vi "Game of Life.vi"() -> ()   [LabVIEW 2021, in "Game of Life.lvlib"]
doc: "InstrumentStudio plug-in example that displays Conway's Game of Life simulation in a graph."
uses:
  Game of Life.lvlib
  <vilib>/Plug-In SDKs/InstrumentStudio/Plugin Events Enum.ctl
  Helpers/Data Cluster.ctl
  Helpers/Configuration.ctl
  Queue Driver/Queue Operations.ctl
  Queue Driver/Queue State and Data.ctl
  User Event Driver/User Event Operations.ctl
  Helpers/Graph Elements.ctl
  <vilib>/Utility/error.llb/DialogType.ctl
  <vilib>/Utility/error.llb/Error Cluster From Error Code.vi
  <vilib>/ErrorRing/Error Ring.xnode
  <vilib>/Plug-In SDKs/InstrumentStudio/Plugin Session.lvclass
  <vilib>/Plug-In SDKs/InstrumentStudio/InstrumentStudio Plugin SDK.lvlib
  Queue Driver/Queue Driver.lvlib
  User Event Driver/User Event Driver.lvlib
panel:
  in  "Tab Control":enum32{"Game Panel", "Events"}(tab)
  in  "width":u32=100 caption="Board width" min=5 max=1000 step=1
  in  "height":u32=100 caption="Board height" min=5 max=1000 step=1
  in  "update interval":u32=500 caption="Update interval (msec)" min=100 max=2000 step=100
  out "generation":u32 caption="Generation"
  out "game of life":T1(graph)
  in  "Start/Stop":bool
  in  "Log Events?":bool caption="Enable Logging"
  out "Event Record":i32(listbox)=-1
  out "Log file directory":path
  in  "Session Id":u64
  # "When logging is enabled, a log file will be generated in the specified \ndirectory after the front panel is closed."
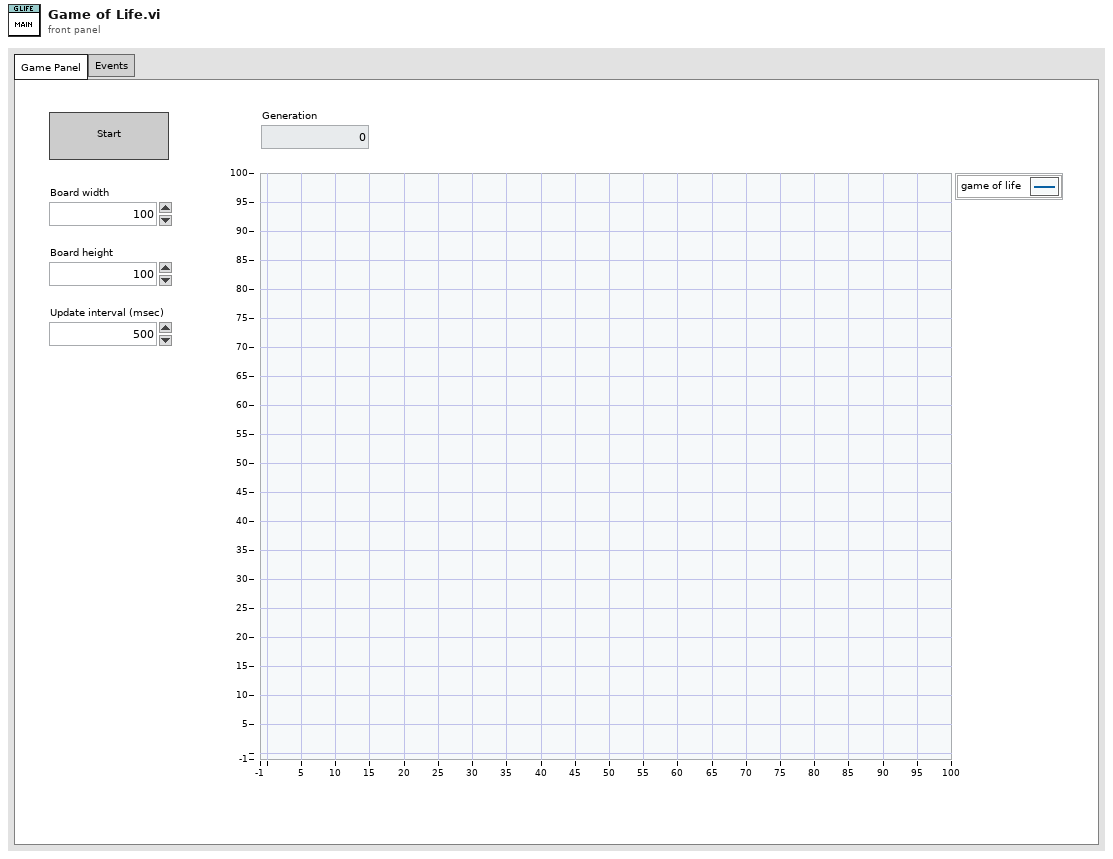
[diagram p1: front panel]
types:
  T1 = typedef "Game of Life.lvlib/Graph Elements.ctl" = cluster{"x data":dbl[], "y data":dbl[]}
  T2 = typedef "Game of Life.lvlib/User Event Driver.lvlib/User Event Operations.ctl" = enum16{"Create", "Destroy", "Get Reference", "Generate"}
  T3 = typedef "Game of Life.lvlib/Queue Driver.lvlib/Queue State and Data.ctl" = cluster{"state":string, "data":variant}
  T4 = typedef "Game of Life.lvlib/Queue Driver.lvlib/Queue Operations.ctl" = enum16{"Create Q", "Enqueue", "Enqueue N", "Enstack", "Enstack N", "Dequeue", "Flush", "Release"}
  T5 = typedef "Game of Life.lvlib/Data Cluster.ctl" = cluster{"configuration":T6, "generation":u32, "cells":bool[][], "event records":string[], "running?":bool, "board update time":timestamp}
  T6 = typedef "Game of Life.lvlib/Configuration.ctl" = cluster{"height":u32, "width":u32, "interval":u32, "log path":string, "log events?":bool}
  T7 = typedef "InstrumentStudio Plugin SDK.lvlib/Plugin Events Enum.ctl" = enum32{"Shutdown", "Project Saved", "Stop All Outputs", "Generic Message", "Active Pin Map Changed", "Selected Sites Changed"}
  T8 = typedef "InstrumentStudio Plugin SDK.lvlib/Event Registration Refnum.ctl" = refnum<event-registration>
  T9 = cluster{"Event Refnum":T8, "Event Registration Refnum":refnum<event-registration>}
  T10 = enum8{"Enabled", "Disabled", "Disabled and Grayed Out"}
  T11 = typedef "DialogType.ctl" = u16
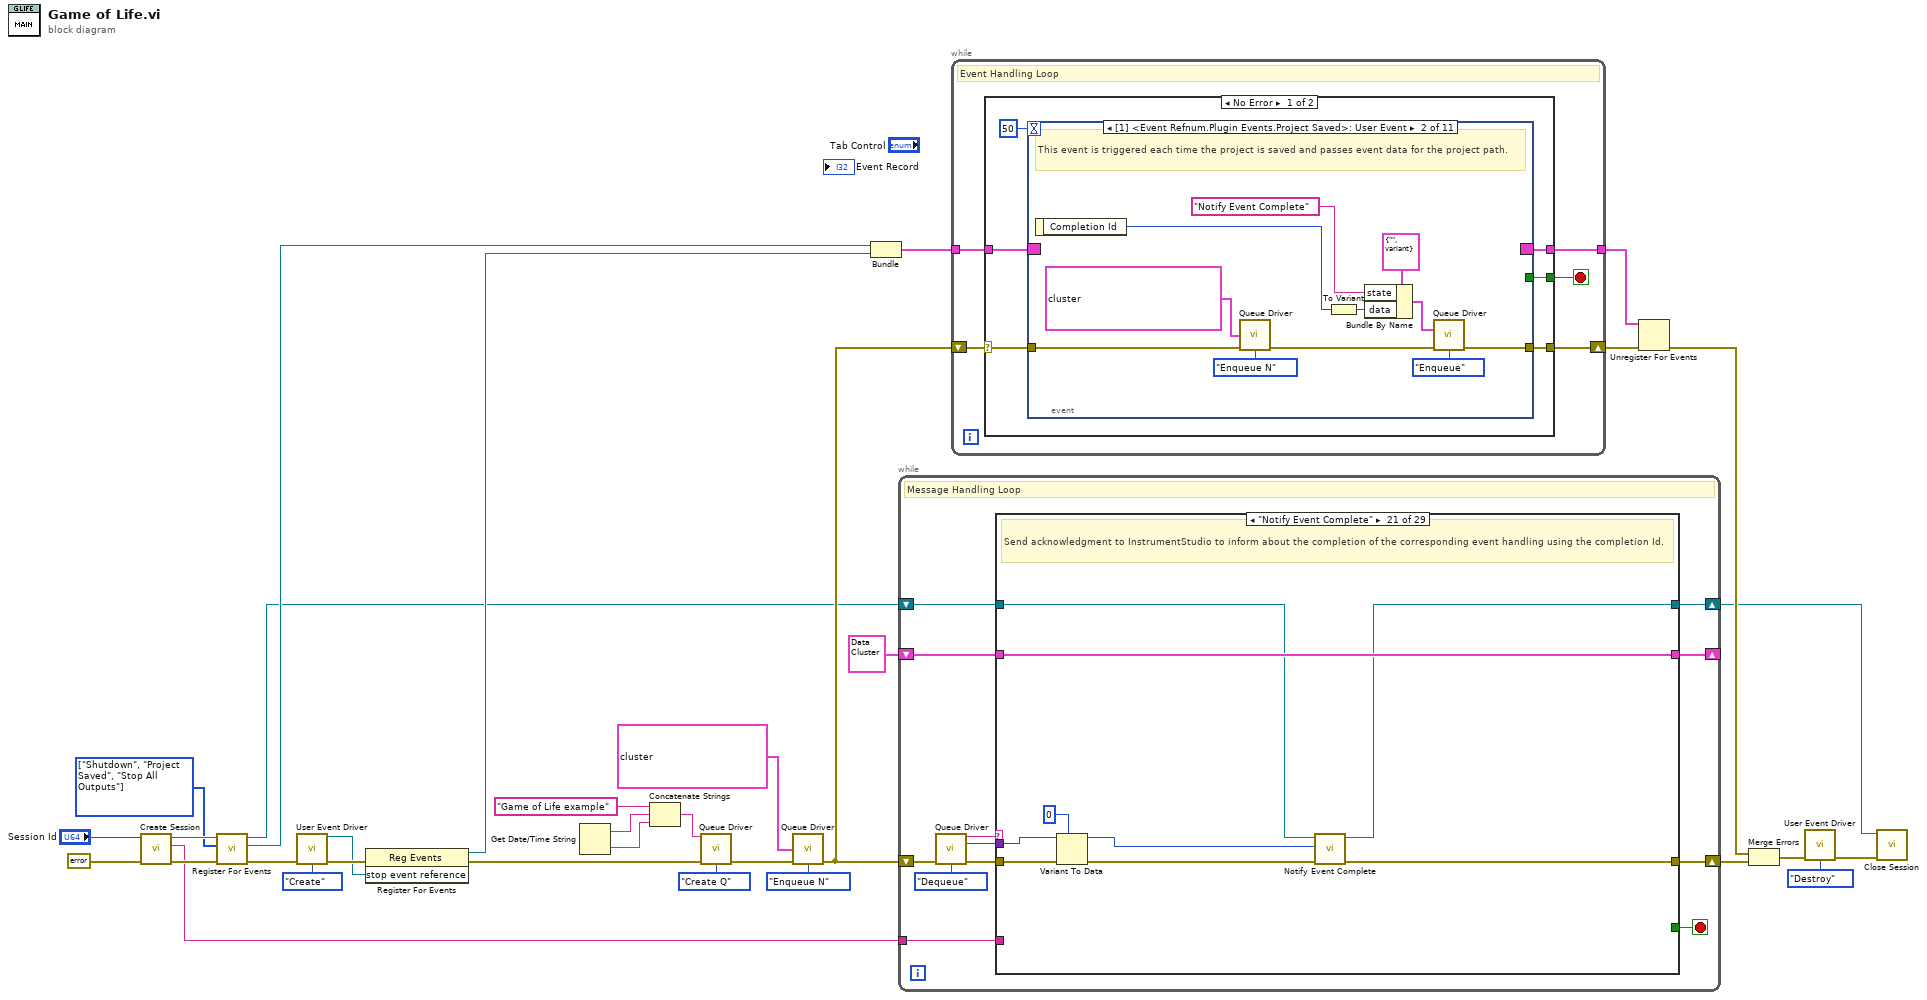
[diagram p0: block diagram]
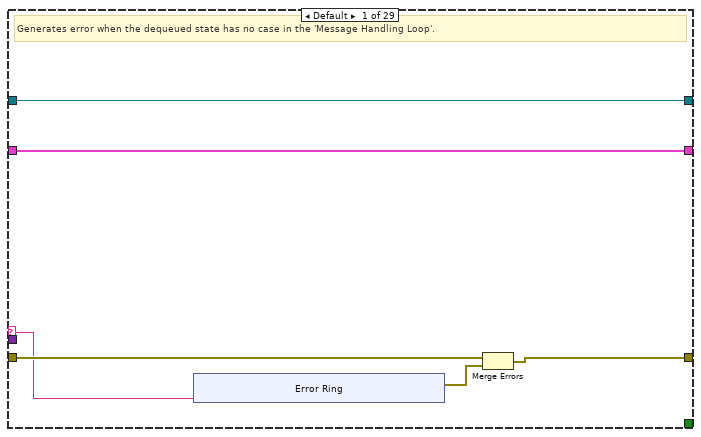
[diagram p2: hidden frame]
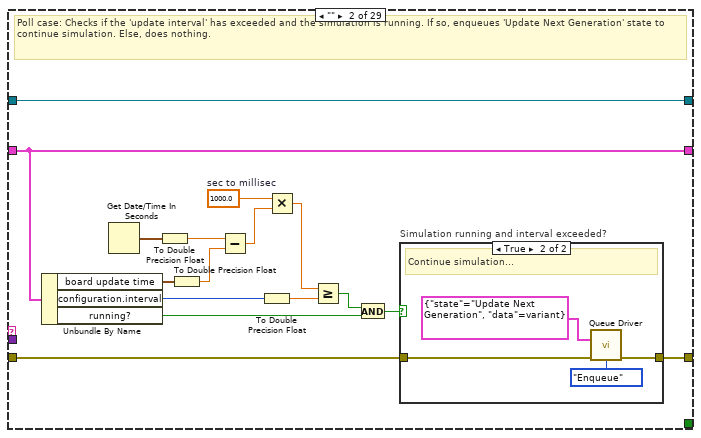
[diagram p3: hidden frame]
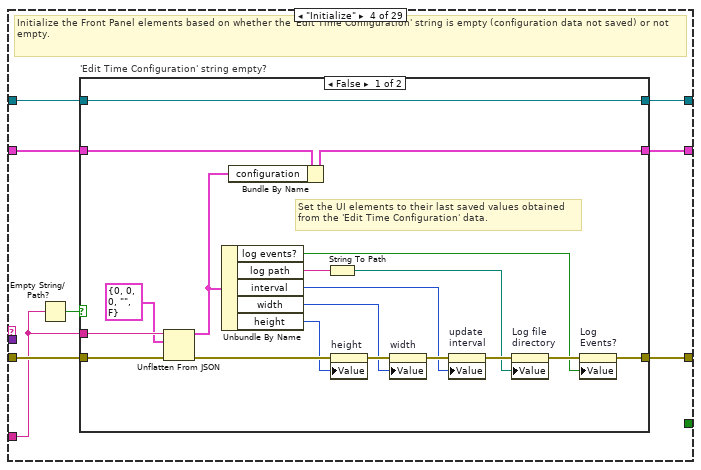
[diagram p6: hidden frame]
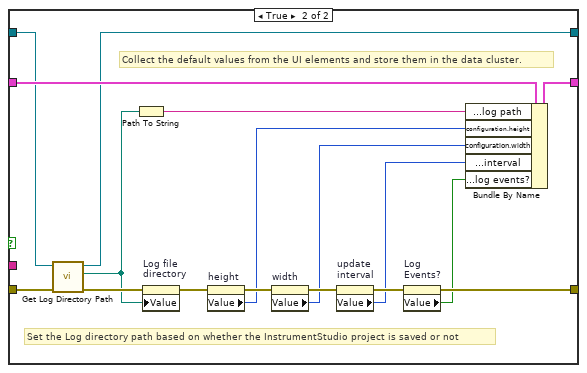
[diagram p7: hidden frame]
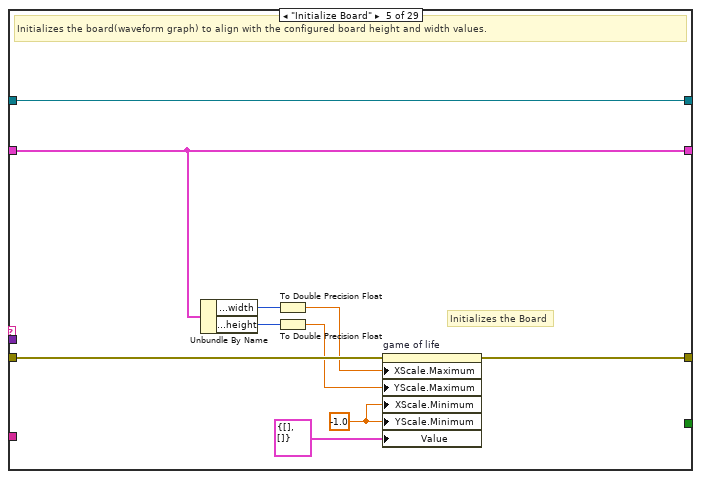
[diagram p8: hidden frame]
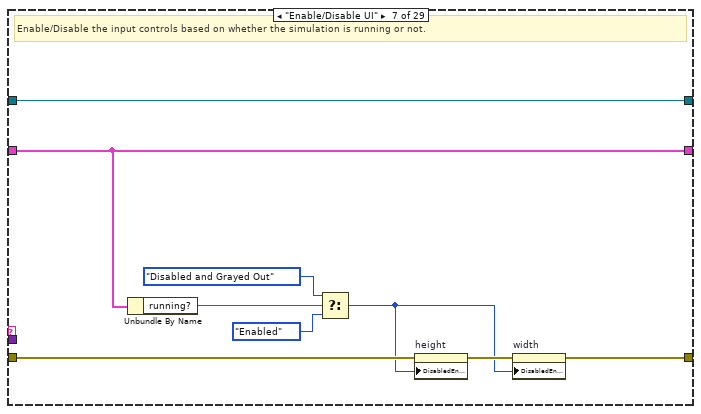
[diagram p10: hidden frame]
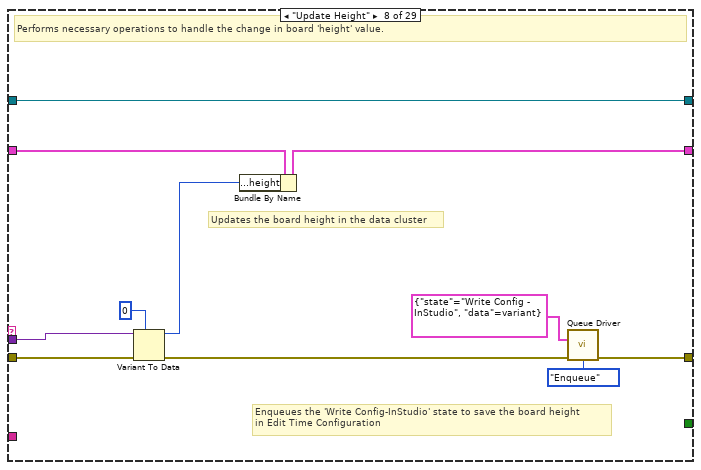
[diagram p11: hidden frame]
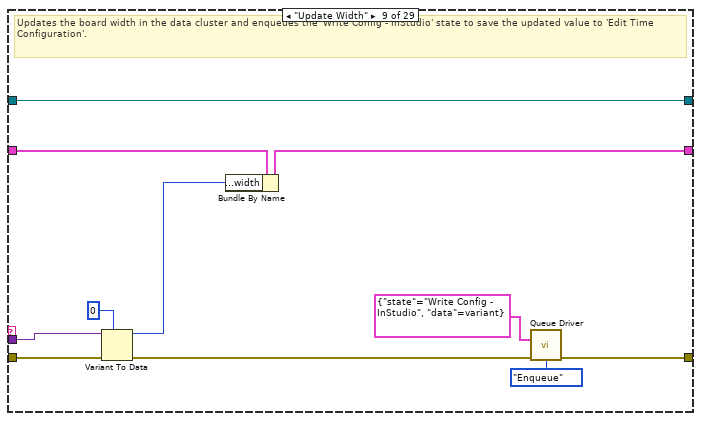
[diagram p12: hidden frame]
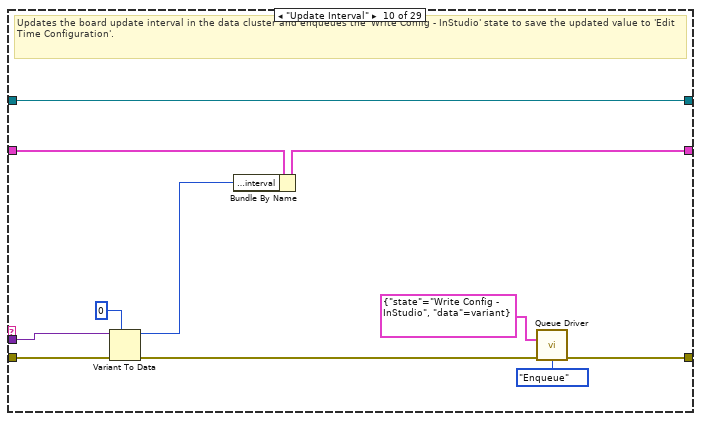
[diagram p13: hidden frame]
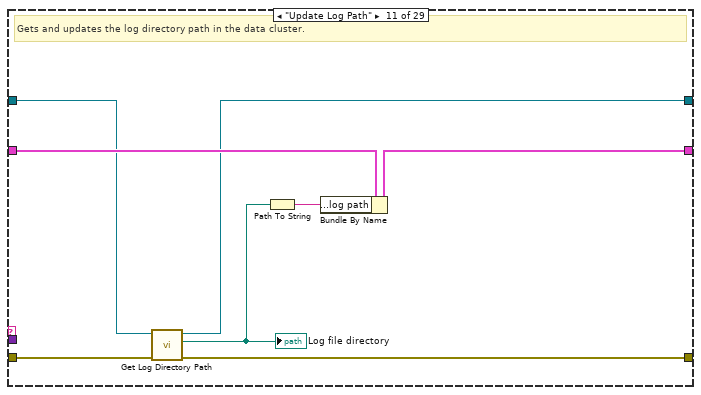
[diagram p14: hidden frame]
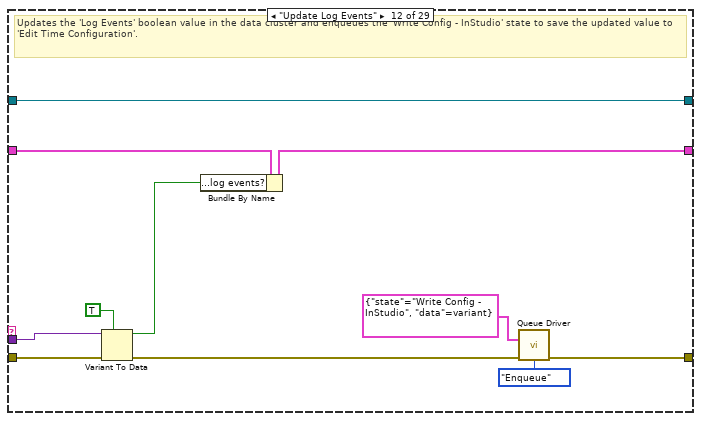
[diagram p15: hidden frame]
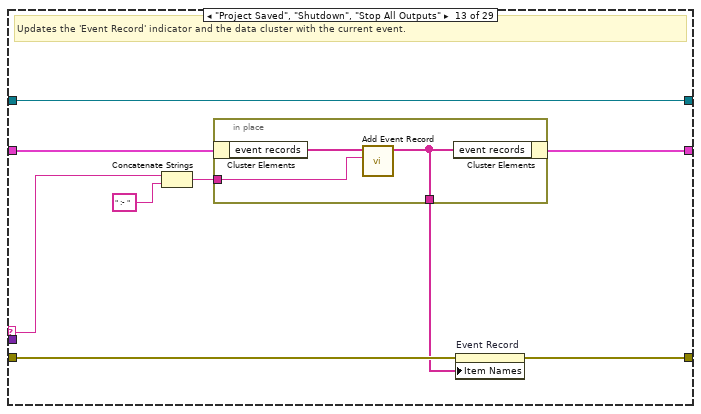
[diagram p16: hidden frame]
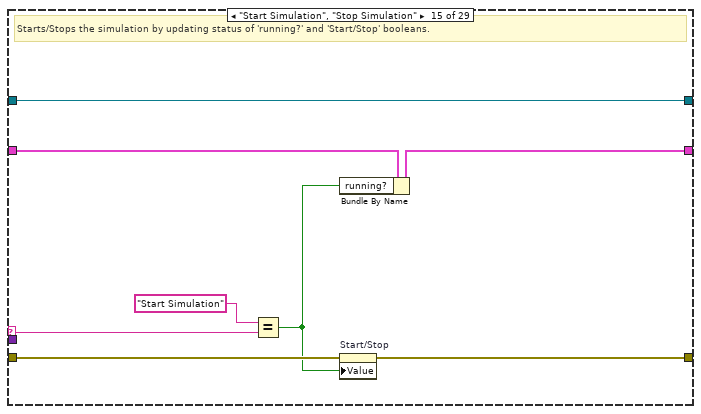
[diagram p18: hidden frame]
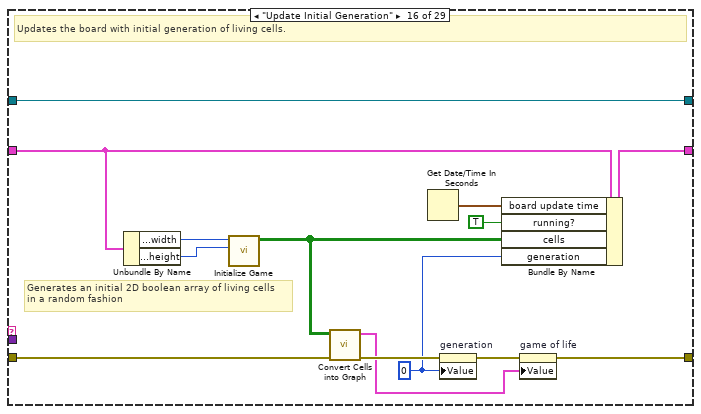
[diagram p19: hidden frame]
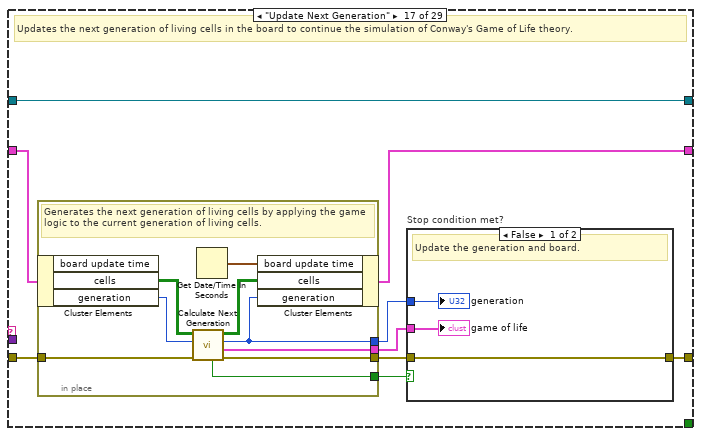
[diagram p20: hidden frame]
diagram:
  w22 = T7[] [enum."Shutdown", enum."Project Saved", enum."Stop All Outputs"] items=["Shutdown", "Project Saved", "Stop All Outputs", "Generic Message", "Active Pin Map Changed", "Selected Sites Changed"] ("Events To Register")
  n1 = call <vilib>:"Create Session.vi"("error in (no error)"=errorcluster {"status"=FALSE, "code"=0, "source"=""}, "Session Id"="Session Id") -> ("error out"=w9:errorcluster, "Edit Time Configuration"=w1:string, "Session out"=w23:refnum<class "Plugin Session.lvclass">)  [unwired: 5 in, 2 out]
  n2 = call <vilib>:"Register For Events.vi"("error in (no error)"=w9, "Events To Register"=w22, "Session in"=w23) -> ("error out"=w8:errorcluster, "Event Refnum"=w21:T8, "Session out"=w3:refnum<class "Plugin Session.lvclass">)  [unwired: 6 in]
  n3 = call "User Event Driver.vi"("error in"=w8, "user event operation"=User_Event_Operations."Create" ("LV2 Operation")) -> ("stop event reference"=w6:refnum<user-event>, "error out"=w7:errorcluster)  [unwired: 12 in]
  n4 = register-events(error in=w7, w6) -> (reference out=w20:refnum<event-registration>, error out=w18:errorcluster)  [unwired: 1 in]
  n5 = Get Date/Time String() -> (date string=w31:string, time string=w32:string)  [unwired: 3 in]
  n6 = Concatenate Strings("Game of Life example" ("Name"), w31, w32) -> (w27:string)
  n7 = call "Queue Driver.vi"("queue name"=w27, "error in"=w18, "queue operation"=Queue_Operations."Create Q" ("Queue Operations")) -> ("error out"=w28:errorcluster)  [unwired: 10 in, 2 out]
  n8 = call "Queue Driver.vi"("array of state and data"=T3[] [{"state"="Initialize", "data"=variant}, {"state"="Initialize Board", "data"=variant}, {"state"="Enable/Disable UI", "data"=variant}] ("Array of State and Data"), "error in"=w28, "queue operation"=Queue_Operations."Enqueue N" ("Queue Operations")) -> ("error out"=w4:errorcluster)  [unwired: 10 in, 2 out]
  n9 = Bundle("Event Refnum"=w21, "Event Registration Refnum"=w20) -> (w19:T9)  [unwired: 1 in]
  n10 = while {
    shift-right: [w37] -> w14
    shift-left: w4 -> [w45]
    shift-right: [w42] -> _
    shift-left: T5 {"configuration"={"height"=0, "width"=0, "interval"=0, "log path"="", "log events?"=FALSE}, "generation"=0, "cells"=[], "event records"=[], "running?"=FALSE, "board update time"=timestamp(0 s since 1904-01-01)} ("Data") -> [w38]
    shift-right: [w41] -> w15
    shift-left: w3 -> [w40]
    tunnel: w1 -> [w34]
    stop <- w39 stop-if-true
    # "Message Handling Loop"
    n11 = call "Queue Driver.vi"("error in"=w45, "queue operation"=Queue_Operations."Dequeue" ("Queue Operations")) -> ("dequeued state"=w36:string, "dequeued data"=w35:variant, "error out"=w44:errorcluster)  [unwired: 11 in]
    n12 = case shown="\"Notify Event Complete\"" w36 {
      selector: w36 -> [w46 _ _ _ _ _ _ _ _ _ _ _ w204 _ w217 _ _ _ _ _ _ _ _ _ _ _ _ _ _]
      tunnel: w40 -> [w47 w74 w80 w85 w136 w137 w148 w159 w170 w181 w183 w200 w201 w213 w223 w237 w246 w263 w267 w275 w282 w290 w298 w306 w321 w339 w343 w352 w368]
      tunnel: [w49 w73 w82 w89 w133 w139 w140 w150 w160 w171 w189 w190 w208 w215 w221 w234 w243 w265 w270 w278 w287 w292 w297 w308 w315 w335 w345 w347 w361] -> w37
      tunnel: w44 -> [w51 w72 w82 w90 w135 w139 w147 w158 w169 w180 w185 w199 w209 w215 w222 w233 w245 w265 w271 w280 w289 w292 w299 w308 w312 w331 w345 w348 w367]
      tunnel: w38 -> [w48 w63 w81 w88 w128 w138 w145 w155 w166 w177 w187 w195 w203 w214 w219 w230 w244 w264 w269 w276 w288 w291 w296 w307 w310 w326 w344 w353 w369]
      tunnel: [w48 w63 w81 w87 w128 w138 w145 w154 w165 w176 w186 w194 w202 w214 w220 w235 w242 w264 w269 w276 w288 w291 w296 w307 w309 w325 w344 w353 w369] -> w42
      tunnel: [w47 w74 w80 w84 w136 w137 w148 w159 w170 w181 w182 w200 w201 w213 w223 w237 w246 w263 w266 w274 w281 w290 w298 w306 w321 w339 w343 w352 w368] -> w41
      tunnel: [_ _ _ _ _ _ _ _ _ _ _ _ _ _ _ _ _ _ _ _ _ _ _ _ _ _ _ _ TRUE] -> w39
      tunnel: w35 -> [_ _ _ _ _ _ _ w156 w167 w178 _ w197 _ _ _ _ _ _ _ _ w285 _ _ _ _ w334 _ _ _]
      tunnel: w34 -> [_ _ _ w83 _ _ _ _ _ _ _ _ _ _ _ _ _ _ _ _ _ _ _ _ _ _ _ _ _]
      frame Default {
        # "Generates error when the dequeued state has no case in the 'Message Handling Loop'."
        n13 = xnode "Error Ring"("parameter 0"=w46) -> ("error out"=w50:errorcluster)
        n14 = Merge Errors(w51, w50) -> (w49:errorcluster)
      }
      frame "" {
        w69 = 1000.0  # sec to millisec
        # "Poll case: Checks if the 'update interval' has exceeded and the simulation is running. If so, enqueues 'Update Next Generation' state to continue simulation. Else, does nothing."
        n15 = Unbundle By Name(w63) -> ("board update time"=w65:timestamp, "configuration.interval"=w60:u32, "running?"=w62:bool)
        n16 = Get Date/Time In Seconds() -> (seconds since 1Jan1904=w64:timestamp)
        n17 = To Double Precision Float(number=w64) -> (double precision float=w70:dbl)
        n18 = To Double Precision Float(number=w65) -> (double precision float=w71:dbl)
        n19 = Subtract(x=w70, y=w71) -> (x-y=w68:dbl)
        n20 = To Double Precision Float(number=w60) -> (double precision float=w66:dbl)
        n21 = Multiply(x=w69, y=w68) -> (x*y=w67:dbl)
        n22 = Greater Or Equal?(x=w67, y=w66) -> (x >= y?=w61:bool)
        n23 = And(x=w61, y=w62) -> (x .and. y?=w59:bool)
        n24 = case "Simulation running and interval exceeded?" shown="True" w59 {
          tunnel: w72 -> [w75 w78]
          tunnel: [w75 w77] -> w73
          frame False {
            # "Pass"
          }
          frame True {
            # "Continue simulation..."
            n25 = call "Queue Driver.vi"("state and data"=T3 {"state"="Update Next Generation", "data"=variant} ("State and Data"), "error in"=w78, "queue operation"=Queue_Operations."Enqueue" ("Queue Operations")) -> ("error out"=w77:errorcluster)  [unwired: 10 in, 2 out]
          }
        }
      }
      frame "*****Initialization*****" {
      }
      frame "Initialize" {
        # "Initialize the Front Panel elements based on whether the 'Edit Time Configuration' string is empty (configuration data not saved) or not empty."
        n26 = Empty String/Path?(string/path=w83) -> (empty?=w86:bool)
        n27 = case "'Edit Time Configuration' string empty?" shown="False" w86 {
          tunnel: w90 -> [w97 w126]
          tunnel: [w108 w115] -> w89
          tunnel: w88 -> [w100 w120]
          tunnel: [w99 w119] -> w87
          tunnel: w85 -> [w93 w113]
          tunnel: [w93 w111] -> w84
          tunnel: w83 -> [w92 _]
          frame False {
            # "Set the UI elements to their last saved values obtained\nfrom the 'Edit Time Configuration' data."
            n28 = Unflatten From JSON(JSON string=w92, type and defaults=T6 {"height"=0, "width"=0, "interval"=0, "log path"="", "log events?"=FALSE} ("Configuration"), error in (no error)=w97) -> (value=w95:T6, error out=w96:errorcluster)  [unwired: 4 in]
            n29 = Unbundle By Name(w95) -> ("log events?"=w101:bool, "log path"=w104:string, "interval"=w103:u32, "width"=w102:u32, "height"=w94:u32)
            n30 = Bundle By Name(cluster=w100, "configuration"=w95) -> (w99:T5)
            n31 = String To Path(string=w104) -> (path=w98:path)
            n32 = property on="height" class="DigNum (strict)"(error in=w96, "Value"=w94) -> (error out=w105:errorcluster)  [unwired: 1 in, 1 out]
            n33 = property on="width" class="DigNum (strict)"(error in=w105, "Value"=w102) -> (error out=w107:errorcluster)  [unwired: 1 in, 1 out]
            n34 = property on="update\ninterval" class="DigNum (strict)"(error in=w107, "Value"=w103) -> (error out=w106:errorcluster)  [unwired: 1 in, 1 out]
            n35 = property on="Log file\ndirectory" class="Path"(error in=w106, "Value"=w98) -> (error out=w109:errorcluster)  [unwired: 1 in, 1 out]
            n36 = property on="Log\nEvents?" class="Bool (strict)"(error in=w109, "Value"=w101) -> (error out=w108:errorcluster)  [unwired: 1 in, 1 out]
          }
          frame True {
            # "Set the Log directory path based on whether the InstrumentStudio project is saved or not"
            # "Collect the default values from the UI elements and store them in the data cluster."
            n37 = call "Get Log Directory Path.vi"("error in"=w126, "session in"=w113) -> ("error out"=w121:errorcluster, "log directory path"=w110:path, "session out"=w111:refnum<class "Plugin Session.lvclass">)  [unwired: 7 in]
            n38 = Path To String(path=w110) -> (string=w112:string)
            n39 = property on="Log file\ndirectory" class="Path"(error in=w121, "Value"=w110) -> (error out=w122:errorcluster)  [unwired: 1 in, 1 out]
            n40 = property on="height" class="DigNum (strict)"(error in=w122) -> (error out=w124:errorcluster, "Value"=w118:u32)  [unwired: 1 in, 1 out]
            n41 = property on="width" class="DigNum (strict)"(error in=w124) -> (error out=w125:errorcluster, "Value"=w117:u32)  [unwired: 1 in, 1 out]
            n42 = property on="update\ninterval" class="DigNum (strict)"(error in=w125) -> (error out=w123:errorcluster, "Value"=w116:u32)  [unwired: 1 in, 1 out]
            n43 = property on="Log\nEvents?" class="Bool (strict)"(error in=w123) -> (error out=w115:errorcluster, "Value"=w114:bool)  [unwired: 1 in, 1 out]
            n44 = Bundle By Name(cluster=w120, "configuration.log path"=w112, "configuration.height"=w118, "configuration.width"=w117, "configuration.interval"=w116, "configuration.log events?"=w114) -> (w119:T5)
          }
        }
      }
      frame "Initialize Board" {
        w134 = -1.0 ("Y Scale.Range:Minimum")
        # "Initializes the Board"
        # "Initializes the board(waveform graph) to align with the configured board height and width values."
        n45 = Unbundle By Name(w128) -> ("configuration.width"=w132:u32, "configuration.height"=w131:u32)
        n46 = To Double Precision Float(number=w132) -> (double precision float=w130:dbl)
        n47 = To Double Precision Float(number=w131) -> (double precision float=w129:dbl)
        n48 = property on="game of life" class="XYGraph (strict)"(error in=w135, "XScale.Maximum"=w130, "YScale.Maximum"=w129, "XScale.Minimum"=w134, "YScale.Minimum"=w134, "Value"=T1 {"x data"=[], "y data"=[]} ("game of life")) -> (error out=w133:errorcluster)  [unwired: 1 in, 1 out]
      }
      frame "*****Front Panel Updates*****" {
      }
      frame "Enable/Disable UI" {
        # "Enable/Disable the input controls based on whether the simulation is running or not."
        n49 = Unbundle By Name(w145) -> ("running?"=w144:bool)
        n50 = Select(t=T10."Disabled and Grayed Out", s=w144, f=T10."Enabled" ("Disabled")) -> (s? t:f=w141:T10)
        n51 = property on="height" class="DigNum (strict)"(error in=w147, "DisabledEnum"=w141) -> (error out=w146:errorcluster)  [unwired: 1 in, 1 out]
        n52 = property on="width" class="DigNum (strict)"(error in=w146, "DisabledEnum"=w141) -> (error out=w140:errorcluster)  [unwired: 1 in, 1 out]
      }
      frame "Update Height" {
        # "Enqueues the 'Write Config-InStudio' state to save the board height\nin Edit Time Configuration"
        # "Updates the board height in the data cluster"
        # "Performs necessary operations to handle the change in board 'height' value."
        n53 = Variant To Data(error in=w158, type=u32 0, Variant=w156) -> (data=w153:u32, error out=w149:errorcluster)
        n54 = Bundle By Name(cluster=w155, "configuration.height"=w153) -> (w154:T5)
        n55 = call "Queue Driver.vi"("state and data"=T3 {"state"="Write Config - InStudio", "data"=variant} ("State and Data"), "error in"=w149, "queue operation"=Queue_Operations."Enqueue" ("Queue Operations")) -> ("error out"=w150:errorcluster)  [unwired: 10 in, 2 out]
      }
      frame "Update Width" {
        # "Updates the board width in the data cluster and enqueues the 'Write Config - InStudio' state to save the updated value to 'Edit Time Configuration'."
        n56 = Variant To Data(error in=w169, type=u32 0, Variant=w167) -> (data=w164:u32, error out=w161:errorcluster)
        n57 = Bundle By Name(cluster=w166, "configuration.width"=w164) -> (w165:T5)
        n58 = call "Queue Driver.vi"("state and data"=T3 {"state"="Write Config - InStudio", "data"=variant} ("State and Data"), "error in"=w161, "queue operation"=Queue_Operations."Enqueue" ("Queue Operations")) -> ("error out"=w160:errorcluster)  [unwired: 10 in, 2 out]
      }
      frame "Update Interval" {
        # "Updates the board update interval in the data cluster and enqueues the 'Write Config - InStudio' state to save the updated value to 'Edit Time Configuration'."
        n59 = Variant To Data(error in=w180, type=u32 0, Variant=w178) -> (data=w175:u32, error out=w172:errorcluster)
        n60 = Bundle By Name(cluster=w177, "configuration.interval"=w175) -> (w176:T5)
        n61 = call "Queue Driver.vi"("state and data"=T3 {"state"="Write Config - InStudio", "data"=variant} ("State and Data"), "error in"=w172, "queue operation"=Queue_Operations."Enqueue" ("Queue Operations")) -> ("error out"=w171:errorcluster)  [unwired: 10 in, 2 out]
      }
      frame "Update Log Path" {
        # "Gets and updates the log directory path in the data cluster."
        n62 = call "Get Log Directory Path.vi"("error in"=w185, "session in"=w183) -> ("error out"=w189:errorcluster, "log directory path"=w184:path, "session out"=w182:refnum<class "Plugin Session.lvclass">)  [unwired: 7 in]
        "Log file directory" <- w184
        n63 = Path To String(path=w184) -> (string=w188:string)
        n64 = Bundle By Name(cluster=w187, "configuration.log path"=w188) -> (w186:T5)
      }
      frame "Update Log Events" {
        # "Updates the 'Log Events' boolean value in the data cluster and enqueues the 'Write Config - InStudio' state to save the updated value to 'Edit Time Configuration'."
        n65 = Variant To Data(error in=w199, type=TRUE, Variant=w197) -> (data=w196:bool, error out=w191:errorcluster)
        n66 = Bundle By Name(cluster=w195, "configuration.log events?"=w196) -> (w194:T5)
        n67 = call "Queue Driver.vi"("state and data"=T3 {"state"="Write Config - InStudio", "data"=variant} ("State and Data"), "error in"=w191, "queue operation"=Queue_Operations."Enqueue" ("Queue Operations")) -> ("error out"=w190:errorcluster)  [unwired: 10 in, 2 out]
      }
      frame "Project Saved", "Shutdown", "Stop All Outputs" {
        # "Updates the 'Event Record' indicator and the data cluster with the current event."
        n68 = Concatenate Strings(w204, " :- " ("string")) -> (w207:string)
        n69 = in-place {
          in-place-border: w207 -> [w212]
          in-place-border: [w210] -> w206
          n70 = in-place-cluster #1(w203) -> ("event records"=w211:string[])
          n71 = call "Add Event Record.vi"("event tag"=w212, "event records in"=w211) -> ("event records out"=w210:string[])  [unwired: 9 in]
          n72 = in-place-cluster #1("event records"=w210) -> (w202:T5)
        }
        n73 = property on="Event Record" class="LstBox (strict)"(error in=w209, "Item Names"=w206) -> (error out=w208:errorcluster)  [unwired: 1 in, 1 out]
      }
      frame "*****Implementation Logic*****" {
      }
      frame "Start Simulation", "Stop Simulation" {
        # "Starts/Stops the simulation by updating status of 'running?' and 'Start/Stop' booleans."
        n74 = Equal?(x="Start Simulation" ("y"), y=w217) -> (x = y?=w216:bool)
        n75 = Bundle By Name(cluster=w219, "running?"=w216) -> (w220:T5)
        n76 = property on="Start/Stop" class="Bool (strict)"(error in=w222, "Value"=w216) -> (error out=w221:errorcluster)  [unwired: 1 in, 1 out]
      }
      frame "Update Initial Generation" {
        w225 = u32 0 ("Generation")
        # "Generates an initial 2D boolean array of living cells\nin a random fashion"
        # "Updates the board with initial generation of living cells."
        n77 = Unbundle By Name(w230) -> ("configuration.width"=w236:u32, "configuration.height"=w229:u32)
        n78 = call "Initialize Game.vi"("height"=w229, "width"=w236) -> ("living cells"=w224:bool[][])  [unwired: 9 in]
        n79 = call "Convert Cells into Graph.vi"("error in"=w233, "cells in"=w224) -> ("error out"=w232:errorcluster, "graph elements"=w226:T1)  [unwired: 8 in]
        n80 = Get Date/Time In Seconds() -> (seconds since 1Jan1904=w228:timestamp)
        n81 = property on="generation" class="DigNum (strict)"(error in=w232, "Value"=w225) -> (error out=w231:errorcluster)  [unwired: 1 in, 1 out]
        n82 = Bundle By Name(cluster=w230, "board update time"=w228, "running?"=TRUE, "cells"=w224, "generation"=w225) -> (w235:T5)
        n83 = property on="game of life" class="XYGraph (strict)"(error in=w231, "Value"=w226) -> (error out=w234:errorcluster)  [unwired: 1 in, 1 out]
      }
      frame "Update Next Generation" {
        # "Updates the next generation of living cells in the board to continue the simulation of Conway's Game of Life theory."
        n84 = in-place {
          in-place-border: w245 -> [w262]
          in-place-border: [w261] -> w241
          in-place-border: [w256] -> w240
          in-place-border: [w257] -> w239
          in-place-border: [w254] -> w238
          # "Generates the next generation of living cells by applying the game logic to the current generation of living cells."
          n85 = in-place-cluster #2(w244) -> ("cells"=w258:bool[][], "generation"=w260:u32)  [unwired: 1 out]
          n86 = call "Calculate Next Generation.vi"("error in"=w262, "generation in"=w260, "cells in"=w258) -> ("error out"=w261:errorcluster, "graph elements"=w257:T1, "generation out"=w256:u32, "cells out"=w259:bool[][], "stop generation?"=w254:bool)  [unwired: 4 in]
          n87 = Get Date/Time In Seconds() -> (seconds since 1Jan1904=w255:timestamp)
          n88 = in-place-cluster #2("board update time"=w255, "cells"=w259, "generation"=w256) -> (w242:T5)
        }
        n89 = case "Stop condition met?" shown="False" w238 {
          tunnel: w241 -> [w249 w252]
          tunnel: [w249 w251] -> w243
          tunnel: w240 -> [w248 _]
          tunnel: w239 -> [w247 _]
          frame False {
            # "Update the generation and board."
            "generation" <- w248
            "game of life" <- w247
          }
          frame True {
            # "Stop the simulation."
            n90 = call "Queue Driver.vi"("array of state and data"=T3[] [{"state"="Stop Simulation", "data"=variant}, {"state"="Enable/Disable UI", "data"=variant}, {"state"="Update Running Flag", "data"=variant}] ("Array of State and Data"), "error in"=w252, "queue operation"=Queue_Operations."Enqueue N" ("Queue Operations")) -> ("error out"=w251:errorcluster)  [unwired: 10 in, 2 out]
          }
        }
      }
      frame "*****InstrumentStudio Interaction*****" {
      }
      frame "Update Running Flag" {
        # "For reference:"
        # "Updates the running flag in InstrumentStudio."
        n91 = Unbundle By Name(w269) -> ("running?"=w268:bool)
        n92 = call <vilib>:"Update Running State.vi"("error in (no error)"=w271, "Is Running"=w268, "Plugin Session in"=w267) -> ("error out"=w270:errorcluster, "Plugin Session out"=w266:refnum<class "Plugin Session.lvclass">)  [unwired: 7 in]
      }
      frame "Write Config - InStudio" {
        # "Saves the configuration values from the data cluster into the 'Edit Time Configuration' value of the current InstrumentStudio session."
        n93 = Unbundle By Name(w276) -> ("configuration"=w273:T6)
        n94 = Flatten To JSON(enable LabVIEW extensions? (T)=FALSE, anything=w273, error in (no error)=w280) -> (JSON string=w277:string, 11:w279:errorcluster)
        n95 = call <vilib>:"Write Edit Time Configuration.vi"("error in (no error)"=w279, "Edit Time Configuration"=w277, "Session in"=w275) -> ("error out"=w278:errorcluster, "Session out"=w274:refnum<class "Plugin Session.lvclass">)  [unwired: 7 in]
      }
      frame "Notify Event Complete" {
        # "Send acknowledgment to InstrumentStudio to inform about the completion of the corresponding event handling using the completion Id."
        n96 = Variant To Data(error in=w289, type=i64 0, Variant=w285) -> (data=w283:i64, error out=w286:errorcluster)
        n97 = call <vilib>:"Notify Event Complete.vi"("error in (no error)"=w286, "Completion Id"=w283, "Session in"=w282) -> ("error out"=w287:errorcluster, "Session out"=w281:refnum<class "Plugin Session.lvclass">)  [unwired: 7 in]
      }
      frame "*****Log Operations*****" {
      }
      frame "Log Events" {
        # "Logs the recorded events to a CSV file if the 'Log Events' check box is enabled."
        n98 = Unbundle By Name(w296) -> ("configuration.log events?"=w293:bool, "configuration.log path"=w295:string, "event records"=w294:string[])
        n99 = case shown="True" w293 {
          tunnel: w299 -> [w300 w305]
          tunnel: [w300 w304] -> w297
          tunnel: w295 -> [_ w303]
          tunnel: w294 -> [_ w302]
          frame False {
          }
          frame True {
            n100 = String To Path(string=w303) -> (path=w301:path)
            n101 = call "Log Events.vi"("error in"=w305, "event records"=w302, "log directory path"=w301) -> ("error out"=w304:errorcluster)  [unwired: 8 in]
          }
        }
      }
      frame "*****Error Handling*****" {
      }
      frame "Error" {
        w320 = T11 0 items=["no dialog", "OK message", "continue or stop message", "OK message + warnings", "continue/stop + warnings"] ("type of dialog (OK msg:1)")
        # "Log error in the 'Event Record'"
        # "Performs the necessary error handling for any error encountered in 'Message Handling Loop'."
        n102 = call <vilib>:"Simple Error Handler.vi"("type of dialog (OK msg:1)"=w320, "error in (no error)"=w312) -> ("error out"=w316:errorcluster, "message"=w314:string)  [unwired: 3 in, 3 out]
        n103 = call "Align Error Message.vi"("message in"=w314) -> ("message out"=w319:string)  [unwired: 10 in]
        n104 = Concatenate Strings(w319, " :- " ("string")) -> (w317:string)
        n105 = in-place {
          in-place-border: w317 -> [w323]
          in-place-border: [w322] -> w311
          n106 = in-place-cluster #3(w310) -> ("event records"=w324:string[])
          n107 = call "Add Event Record.vi"("event tag"=w323, "event records in"=w324) -> ("event records out"=w322:string[])  [unwired: 9 in]
          n108 = in-place-cluster #3("event records"=w322) -> (w309:T5)
        }
        n109 = call <vilib>:"Clear Errors.vi"("error in (no error)"=w316) -> ("error out"=w313:errorcluster)  [unwired: 5 in, 1 out]
        n110 = property on="Event Record" class="LstBox (strict)"(error in=w313, "Item Names"=w311) -> (error out=w315:errorcluster)  [unwired: 1 in, 1 out]
      }
      frame "Event Handler Error" {
        w333 = T11 0 items=["no dialog", "OK message", "continue or stop message", "OK message + warnings", "continue/stop + warnings"] ("type of dialog (OK msg:1)")
        # "Log error in the 'Event Record'"
        # "Performs the necessary error handling for any error encountered in 'Event Handling Loop'."
        n111 = Variant To Data(error in=w331, type=errorcluster {"status"=FALSE, "code"=0, "source"=""} ("error out"), Variant=w334) -> (data=w328:errorcluster, error out=w330:errorcluster)
        n112 = call <vilib>:"Simple Error Handler.vi"("type of dialog (OK msg:1)"=w333, "error in (no error)"=w328) -> ("message"=w332:string)  [unwired: 3 in, 4 out]
        n113 = call "Align Error Message.vi"("message in"=w332) -> ("message out"=w338:string)  [unwired: 10 in]
        n114 = Concatenate Strings(w338, " :- " ("string")) -> (w336:string)
        n115 = in-place {
          in-place-border: w336 -> [w341]
          in-place-border: [w340] -> w327
          n116 = in-place-cluster #4(w326) -> ("event records"=w342:string[])
          n117 = call "Add Event Record.vi"("event tag"=w341, "event records in"=w342) -> ("event records out"=w340:string[])  [unwired: 9 in]
          n118 = in-place-cluster #4("event records"=w340) -> (w325:T5)
        }
        n119 = property on="Event Record" class="LstBox (strict)"(error in=w330, "Item Names"=w327) -> (error out=w335:errorcluster)  [unwired: 1 in, 1 out]
      }
      frame "*****Exit Operations*****" {
      }
      frame "Confirm Quit" {
        # "Displays a pop-up to the user to confirm whether the user is sure about quitting."
        n120 = Two Button Dialog(message="Are you sure you want to quit?", 1:"No, continue" ("F button name (\"Cancel\")"), 2:"Yes, quit" ("T button name (\"OK\")")) -> (T button?=w346:bool)
        n121 = case "Quit execution?" shown="True" w346 {
          tunnel: w348 -> [w354 w356]
          tunnel: [w354 w355] -> w347
          frame False {
            # "Continue..."
          }
          frame True {
            # "Exit the application."
            n122 = call "Queue Driver.vi"("array of state and data"=T3[] [{"state"="Stop Simulation", "data"=variant}, {"state"="Enable/Disable UI", "data"=variant}, {"state"="Update Running Flag", "data"=variant}, {"state"="Log Events", "data"=variant}, {"state"="Exit", "data"=variant}] ("Array of State and Data"), "error in"=w356, "queue operation"=Queue_Operations."Enqueue N" ("Queue Operations")) -> ("error out"=w355:errorcluster)  [unwired: 10 in, 2 out]
          }
        }
      }
      frame "Exit" {
        # "Performs the necessary exit operations."
        n123 = property on="Event Record" class="LstBox (strict)"(error in=w367, "Item Names"=string[] []) -> (error out=w364:errorcluster)  [unwired: 1 in, 1 out]
        n124 = invoke class="VI" method="Default Vals.Reinit All"(error in=w364) -> (error out=w363:errorcluster)  [unwired: 2 in, 2 out]
        n125 = call "User Event Driver.vi"("error in"=w363, "user event operation"=User_Event_Operations."Generate" ("LV2 Operation")) -> ("error out"=w362:errorcluster)  [unwired: 12 in, 1 out]
        n126 = call "Queue Driver.vi"("error in"=w362, "queue operation"=Queue_Operations."Release" ("Queue Operations")) -> ("error out"=w361:errorcluster)  [unwired: 11 in, 2 out]
      }
    }
  }
  n127 = while {
    tunnel: w19 -> [w371]
    shift-right: [w373] -> w17
    shift-left: w4 -> [w374]
    tunnel: [w372] -> w5
    stop <- w370 stop-if-true
    # "Event Handling Loop"
    n128 = case shown="No Error" w374 {
      selector: w374 -> [w380 w460]
      tunnel: [w379 w465] -> w373
      tunnel: [w378 _] -> w372
      tunnel: w371 -> [w377 _]
      tunnel: [w375 _] -> w370
      frame No Error {
        n129 = event shown="[1] <Event Refnum.Plugin Events.Project Saved>: User Event" {
          selector: w377 -> [_ _ _ _ _ _ _ _ _ _ _]
          dyn-events: [_ _ _ _ _ _ _ _ _ _ _] -> w378
          timeout: 50 -> [_ _ _ _ _ _ _ _ _ _ _]
          tunnel: [w381 w384 w394 w407 w409 w417 w425 w433 w441 w444 w455] -> w379
          tunnel: w380 -> [w381 w391 w403 w404 w409 w415 w423 w431 w439 w443 w456]
          tunnel: [_ _ _ _ w408 _ _ _ _ _ _] -> w375
          event Timeout {
            n130 = event-data() -> ()  [unwired: 1 in, 1 out]
          }
          event User Event {
            # "This event is triggered each time the project is saved and passes event data for the project path."
            n131 = event-data() -> ("Completion Id"=w383:i64)  [unwired: 1 in]
            n132 = call "Queue Driver.vi"("array of state and data"=T3[] [{"state"="Project Saved", "data"=variant}, {"state"="Update Log Path", "data"=variant}, {"state"="Write Config - InStudio", "data"=variant}] ("Array of State and Data"), "error in"=w391, "queue operation"=Queue_Operations."Enqueue N" ("Queue Operations")) -> ("error out"=w385:errorcluster)  [unwired: 10 in, 2 out]
            n133 = To Variant(anything=w383) -> (Variant=w388:variant)
            n134 = Bundle By Name(cluster=T3 {"state"="", "data"=variant} ("State and Data"), "state"="Notify Event Complete" ("State"), "data"=w388) -> (w387:T3)
            n135 = call "Queue Driver.vi"("state and data"=w387, "error in"=w385, "queue operation"=Queue_Operations."Enqueue" ("Queue Operations")) -> ("error out"=w384:errorcluster)  [unwired: 10 in, 2 out]
          }
          event User Event {
            # "The Stop All Outputs event is triggered when the 'Stop all outputs' button is pressed on the document toolbar."
            n136 = event-data() -> ("Completion Id"=w393:i64)  [unwired: 1 in]
            n137 = call "Queue Driver.vi"("array of state and data"=T3[] [{"state"="Stop All Outputs", "data"=variant}, {"state"="Stop Simulation", "data"=variant}, {"state"="Enable/Disable UI", "data"=variant}, {"state"="Update Running Flag", "data"=variant}] ("Array of State and Data"), "error in"=w403, "queue operation"=Queue_Operations."Enqueue N" ("Queue Operations")) -> ("error out"=w395:errorcluster)  [unwired: 10 in, 2 out]
            n138 = To Variant(anything=w393) -> (Variant=w399:variant)
            n139 = Bundle By Name(cluster=T3 {"state"="", "data"=variant} ("State and Data"), "state"="Notify Event Complete" ("State"), "data"=w399) -> (w398:T3)
            n140 = call "Queue Driver.vi"("state and data"=w398, "error in"=w395, "queue operation"=Queue_Operations."Enqueue" ("Queue Operations")) -> ("error out"=w394:errorcluster)  [unwired: 10 in, 2 out]
          }
          event User Event; Application Instance Close {
            # "This event doesn't need acknowledgment from plugin"
            # "The Shutdown event is triggered when the document containing the plugin is closed, the project containing the plugin is closed, or the plugin panel is removed from the document using the Edit Layout dialog."
            n141 = event-data() -> ()  [unwired: 1 in, 1 out]
            n142 = call "Queue Driver.vi"("array of state and data"=T3[] [{"state"="Shutdown", "data"=variant}, {"state"="Stop Simulation", "data"=variant}, {"state"="Enable/Disable UI", "data"=variant}, {"state"="Update Running Flag", "data"=variant}, {"state"="Log Events", "data"=variant}, {"state"="Exit", "data"=variant}] ("Array of State and Data"), "error in"=w404, "queue operation"=Queue_Operations."Enqueue N" ("Queue Operations")) -> ("error out"=w407:errorcluster)  [unwired: 10 in, 2 out]
          }
          event User Event {
            w408 = TRUE  # Stop execution
            # "The 'Message Handling Loop' encountered the \"Exit\" state which triggered this event to stop the 'Event Handling Loop'."
            n143 = event-data() -> ()  [unwired: 1 in, 1 out]
          }
          event "height": Value Change {
            # "Captures value change in 'height' and sends data to 'Message Handling Loop'."
            n144 = event-data() -> ("NewVal"=w413:u32)  [unwired: 1 in]
            n145 = To Variant(anything=w413) -> (Variant=w412:variant)
            n146 = Bundle By Name(cluster=T3 {"state"="", "data"=variant} ("State and Data"), "state"="Update Height" ("State"), "data"=w412) -> (w411:T3)
            n147 = call "Queue Driver.vi"("state and data"=w411, "error in"=w415, "queue operation"=Queue_Operations."Enqueue" ("Queue Operations")) -> ("error out"=w417:errorcluster)  [unwired: 10 in, 2 out]
          }
          event "width": Value Change {
            # "Captures value change in 'width' and sends data to 'Message Handling Loop'."
            n148 = event-data() -> ("NewVal"=w420:u32)  [unwired: 1 in]
            n149 = To Variant(anything=w420) -> (Variant=w419:variant)
            n150 = Bundle By Name(cluster=T3 {"state"="", "data"=variant} ("State and Data"), "state"="Update Width" ("State"), "data"=w419) -> (w418:T3)
            n151 = call "Queue Driver.vi"("state and data"=w418, "error in"=w423, "queue operation"=Queue_Operations."Enqueue" ("Queue Operations")) -> ("error out"=w425:errorcluster)  [unwired: 10 in, 2 out]
          }
          event "update interval": Value Change {
            # "Captures value change in 'update interval' and sends data to 'Message Handling Loop'."
            n152 = event-data() -> ("NewVal"=w428:u32)  [unwired: 1 in]
            n153 = To Variant(anything=w428) -> (Variant=w427:variant)
            n154 = Bundle By Name(cluster=T3 {"state"="", "data"=variant} ("State and Data"), "state"="Update Interval" ("State"), "data"=w427) -> (w426:T3)
            n155 = call "Queue Driver.vi"("state and data"=w426, "error in"=w431, "queue operation"=Queue_Operations."Enqueue" ("Queue Operations")) -> ("error out"=w433:errorcluster)  [unwired: 10 in, 2 out]
          }
          event "Log Events?": Value Change {
            # "Captures value change in 'Log Events' and sends data to 'Message Handling Loop'."
            n156 = event-data() -> ("NewVal"=w438:bool)  [unwired: 1 in]
            n157 = To Variant(anything=w438) -> (Variant=w437:variant)
            n158 = Bundle By Name(cluster=T3 {"state"="", "data"=variant} ("State and Data"), "state"="Update Log Events" ("State"), "data"=w437) -> (w436:T3)
            n159 = call "Queue Driver.vi"("state and data"=w436, "error in"=w439, "queue operation"=Queue_Operations."Enqueue" ("Queue Operations")) -> ("error out"=w441:errorcluster)  [unwired: 10 in, 2 out]
          }
          event "Start/Stop": Value Change {
            # "Captures value change in 'Start/Stop' button and enqueues the next state for the'Message Handling Loop' based on the new value of the button."
            n160 = event-data() -> ("NewVal"=w442:bool)  [unwired: 1 in]
            n161 = case shown="True" w442 {
              tunnel: [w446 w449] -> w444
              tunnel: w443 -> [w445 w450]
              frame True {
                n162 = call "Queue Driver.vi"("array of state and data"=T3[] [{"state"="Initialize Board", "data"=variant}, {"state"="Start Simulation", "data"=variant}, {"state"="Enable/Disable UI", "data"=variant}, {"state"="Update Running Flag", "data"=variant}, {"state"="Update Initial Generation", "data"=variant}] ("Array of State and Data"), "error in"=w445, "queue operation"=Queue_Operations."Enqueue N" ("Queue Operations")) -> ("error out"=w446:errorcluster)  [unwired: 10 in, 2 out]
              }
              frame False {
                n163 = call "Queue Driver.vi"("array of state and data"=T3[] [{"state"="Stop Simulation", "data"=variant}, {"state"="Enable/Disable UI", "data"=variant}, {"state"="Update Running Flag", "data"=variant}] ("Array of State and Data"), "error in"=w450, "queue operation"=Queue_Operations."Enqueue N" ("Queue Operations")) -> ("error out"=w449:errorcluster)  [unwired: 10 in, 2 out]
              }
            }
          }
          event Panel Close? {
            # "Send the 'Confirm Quit' message if the user closes the panel of the VI. Discard the event so the 'Confirm Quit' message has a chance to run."
            n164 = event-data() -> ()  [unwired: 1 in, 1 out]
            n165 = call "Queue Driver.vi"("state and data"=T3 {"state"="Confirm Quit", "data"=variant} ("State and Data"), "error in"=w456, "queue operation"=Queue_Operations."Enqueue" ("Queue Operations")) -> ("error out"=w455:errorcluster)  [unwired: 10 in, 2 out]
            n166 = event-data("Discard?"=TRUE) -> ()  [unwired: 1 in, 1 out]
          }
        }
      }
      frame Error {
        n167 = To Variant(anything=w460) -> (Variant=w459:variant)
        n168 = call <vilib>:"Clear Errors.vi"("error in (no error)"=w460) -> ("error out"=w458:errorcluster)  [unwired: 5 in, 1 out]
        n169 = Bundle By Name(cluster=T3 {"state"="", "data"=variant} ("state and data"), "state"="Event Handler Error", "data"=w459) -> (w462:T3)
        n170 = call "Queue Driver.vi"("state and data"=w462, "error in"=w458, "queue operation"=Queue_Operations."Enstack") -> ("error out"=w465:errorcluster)  [unwired: 10 in, 2 out]
      }
    }
  }
  n171 = Unregister For Events(event registration refnum=w5, error in=w17) -> (error out=w16:errorcluster)
  n172 = Merge Errors(w16, w14) -> (w13:errorcluster)
  n173 = call "User Event Driver.vi"("error in"=w13, "user event operation"=User_Event_Operations."Destroy" ("LV2 Operation")) -> ("error out"=w12:errorcluster)  [unwired: 12 in, 1 out]
  n174 = call <vilib>:"Close Session.vi"("error in (no error)"=w12, "Session in"=w15) -> ()  [unwired: 9 in, 1 out]
